vi "Measurement UI.vi"() -> ()   [LabVIEW 2022 SP3, in "PureTone Generation.lvlib"]
uses:
  PureTone Generation.lvlib
panel:
  in  "duration":dbl=1.0 caption="Duration" format="%#_g s"
  in  "offset":dbl caption="Offset" format="%#_g V"
  in  "amplitude":dbl=1.0 caption="Amplitude" min=0.0 max=10.0 step=1.0 format="%#_g V"
  in  "frequency":dbl=1000.0 caption="Frequency" min=1.0 max=100000.0 step=1.0 format="%#_4p Hz"
  in  "DAQmx physical channel":tag caption="DAQmx AO Physical Channel"
  # "PURE TONE GENERATOR"
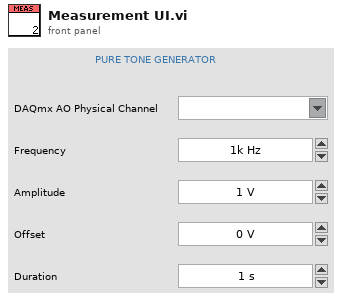
[diagram p1: front panel]
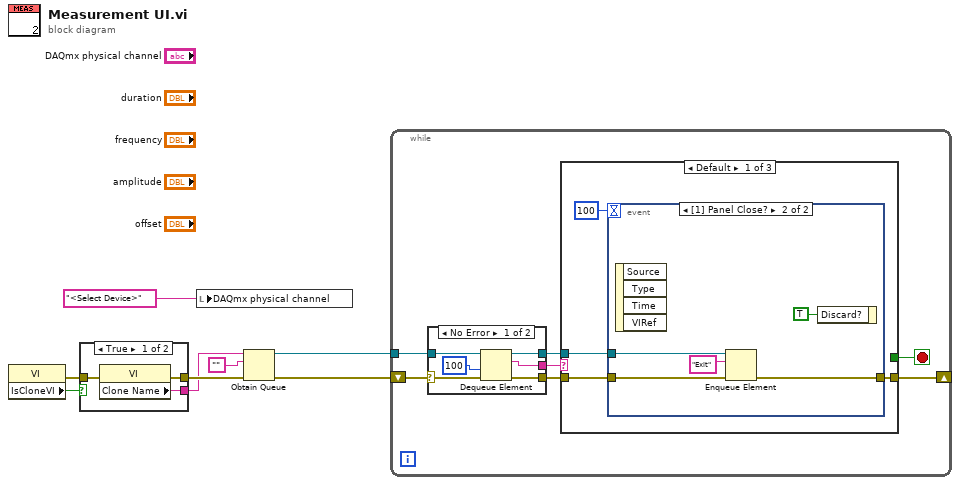
[diagram p0: block diagram]
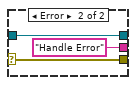
[diagram p2: hidden frame]
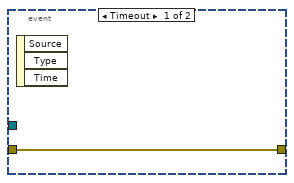
[diagram p3: hidden frame]
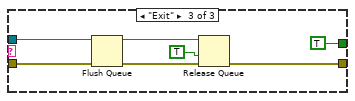
[diagram p5: hidden frame]
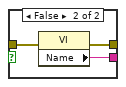
[diagram p6: hidden frame]
diagram:
  n1 = property class="VI"() -> (error out=w2:errorcluster, "IsCloneVI"=w3:bool)  [unwired: 2 in, 1 out]
  n2 = case shown="True" w3 {
    tunnel: [w11 w14] -> w8
    tunnel: [w10 w13] -> w7
    tunnel: w2 -> [w9 w12]
    frame True {
      n3 = property class="VI"(error in=w9) -> (error out=w11:errorcluster, "Clone Name"=w10:string)  [unwired: 1 in, 1 out]
    }
    frame False {
      n4 = property class="VI"(error in=w12) -> (error out=w14:errorcluster, "Name"=w13:string)  [unwired: 1 in, 1 out]
    }
  }
  n5 = local write "DAQmx physical channel"("<Select Device>") -> ()
  n6 = Obtain Queue(name (unnamed)=w7, element data type="", error in (no error)=w8) -> (queue out=w5:refnum<queue>, error out=w6:errorcluster)  [unwired: 2 in, 1 out]
  n7 = while {
    shift-right: [w16] -> _
    shift-left: w6 -> [w21]
    tunnel: w5 -> [w20]
    stop <- w15 stop-if-true
    n8 = case shown="No Error" w21 {
      selector: w21 -> [w27 w30]
      tunnel: [w26 w30] -> w18
      tunnel: w20 -> [w25 w29]
      tunnel: [w24 w29] -> w17
      tunnel: [w23 "Handle Error"] -> w19
      frame No Error {
        n9 = Dequeue Element(queue=w25, timeout in ms (-1)=100, error in (no error)=w27) -> (queue out=w24:refnum<queue>, element=w23:string, error out=w26:errorcluster)  [unwired: 1 out]
      }
      frame Error {
      }
    }
    n10 = case shown="Default" w19 {
      tunnel: w18 -> [w33 w41 w43]
      tunnel: w17 -> [w32 _ w45]
      tunnel: [w31 w41 w44] -> w16
      tunnel: [_ _ TRUE ("force destroy? (F)")] -> w15
      frame Default {
        n11 = event shown="[1] Panel Close?" {
          selector: _ -> [_ _]
          dyn-events: _ -> [_ _]
          timeout: 100 -> [_ _]
          tunnel: w33 -> [w35 w39]
          tunnel: w32 -> [_ w38]
          tunnel: [w35 w36] -> w31
          event Timeout {
            n12 = event-data() -> ()  [unwired: 1 in, 3 out]
          }
          event Panel Close? {
            n13 = event-data() -> ()  [unwired: 1 in, 4 out]
            n14 = Enqueue Element(queue=w38, element="Exit", error in (no error)=w39) -> (error out=w36:errorcluster)  [unwired: 1 in, 2 out]
            n15 = event-data("Discard?"=TRUE) -> ()  [unwired: 1 in, 1 out]
          }
        }
      }
      frame "Handle Error" {
      }
      frame "Exit" {
        n16 = Flush Queue(queue=w45, error in (no error)=w43) -> (queue out=w48:refnum<queue>, error out=w47:errorcluster)  [unwired: 1 out]
        n17 = Release Queue(queue=w48, force destroy? (F)=TRUE, error in (no error)=w47) -> (error out=w44:errorcluster)  [unwired: 2 out]
      }
    }
  }
